vi "Go to IDLE.vi"(8 "error in (no error)":errorcluster, 11 "IDLE in":refnum<class "IDLE.lvclass">) -> (0 "error out":errorcluster, 3 "State Actor.lvclass":refnum<class "State Actor.lvclass">)   [LabVIEW 2021, in "Chef States.lvlib" / "IDLE.lvclass"]
uses:
  IDLE.lvclass
  <vilib>/NI/Actors/State Actor/State Actor/State Actor.lvclass
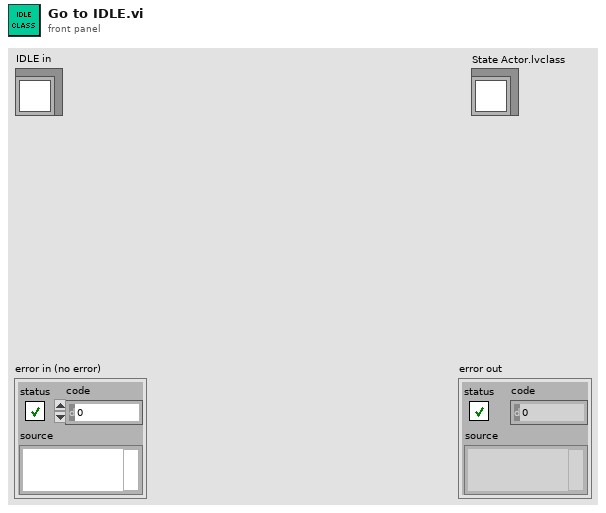
[diagram p1: front panel]
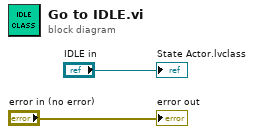
[diagram p0: block diagram]
diagram:
  "error out" <- "error in (no error)"
  "State Actor.lvclass" <- "IDLE in"
